vi "Track FIFO Utilization.vi"(7 "reset":bool, 10 "latch utilization":bool, 11 "samples available":u32) -> (3 "FIFO utilization":T1)   [LabVIEW 2018, in "Streaming FPGA.lvlib"]
doc: "Tracks the minimum and maximum FIFO utilization.\n\nInputs:\n\n<B>samples available</B>: The number of samples available in the FIFO.\n\n<B>reset</B>: A true on this input disables the utilization tracking and sets the outputs to zero (with 2 clock cycles delay). A falling edge on this input starts a new tracking period.\n\n<B>latch utilization</B>: A rising edge on this input updates the outputs (with 1 clock cycle delay) and starts a new tracking period.\n\nOutput:\n\n<B>FIFO utilization</B>: The <B>lowest</B> and <B>highest</B> value provided on the <B>samples available</B> input during the previous tracking period."
uses:
  Streaming FPGA.lvlib
  FIFO Utilization.ctl
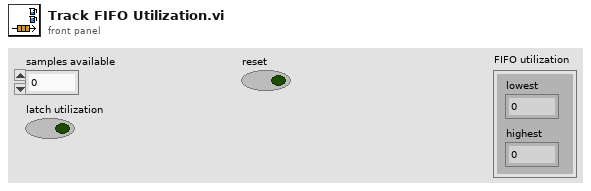
[diagram p1: front panel]
types:
  T1 = typedef "Streaming FPGA.lvlib/FIFO Utilization.ctl" = cluster{"lowest":u32, "highest":u32}
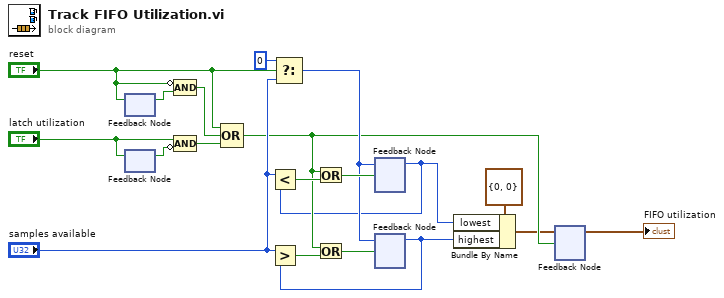
[diagram p0: block diagram]
diagram:
  n1 = feedback #1() -> (w14:bool)  [unwired: 1 in]
  n2 = feedback-in #1("reset") -> ()
  n3 = feedback-in #2("latch utilization") -> ()
  n4 = feedback #2() -> (w19:bool)  [unwired: 1 in]
  n5 = Compound Arithmetic op=AND(invert "reset", w14) -> (w13:bool)
  n6 = Compound Arithmetic op=AND("latch utilization", invert w19) -> (w17:bool)
  n7 = Compound Arithmetic op=OR("reset", w13, w17) -> (w6:bool)
  n8 = Select(t=u32 0, s="reset", f="samples available") -> (s? t:f=w7:u32)
  n9 = feedback #3() -> (w3:u32)  [unwired: 1 in]
  n10 = Less?(x="samples available", y=w3) -> (x < y?=w16:bool)
  n11 = Or(x=w6, y=w16) -> (x .or. y?=w15:bool)
  n12 = feedback-in #3(w7, w15) -> ()
  n13 = feedback #4() -> (w4:u32)  [unwired: 1 in]
  n14 = Greater?(x="samples available", y=w4) -> (0:w9:bool)
  n15 = Or(x=w6, y=w9) -> (x .or. y?=w10:bool)
  n16 = feedback-in #4(w7, w10) -> ()
  n17 = Bundle By Name(cluster=T1 {"lowest"=0, "highest"=0} ("FIFO Utilization"), "lowest"=w3, "highest"=w4) -> (w2:T1)
  n18 = feedback #5() -> (→"FIFO utilization":T1)  [unwired: 1 in]
  n19 = feedback-in #5(w2, w6) -> ()
